vi "Delete Line.vi"(8 "error in":errorcluster, 10 "Active Line Name":string, 11 "dds configuration in":refnum<class "DDS configuration.lvclass">) -> (0 "error out":errorcluster, 2 "deleted line":T1, 3 "dds configuration out":refnum<class "DDS configuration.lvclass">)   [LabVIEW 2014, in "DDS configuration.lvclass"]
uses:
  DDS configuration.lvclass
  Line.ctl
  <vilib>/NI/Tag Bus Module Framework/channel/TBM channel.lvclass
  <vilib>/RTI DDS Toolkit for LabVIEW/Types/RTI DDS Advanced Reader Configuration.ctl
  DDS configuration.lvclass/DDS configuration.ctl
  <vilib>/RTI DDS Toolkit for LabVIEW/Library/LVDDS_library.lvlib
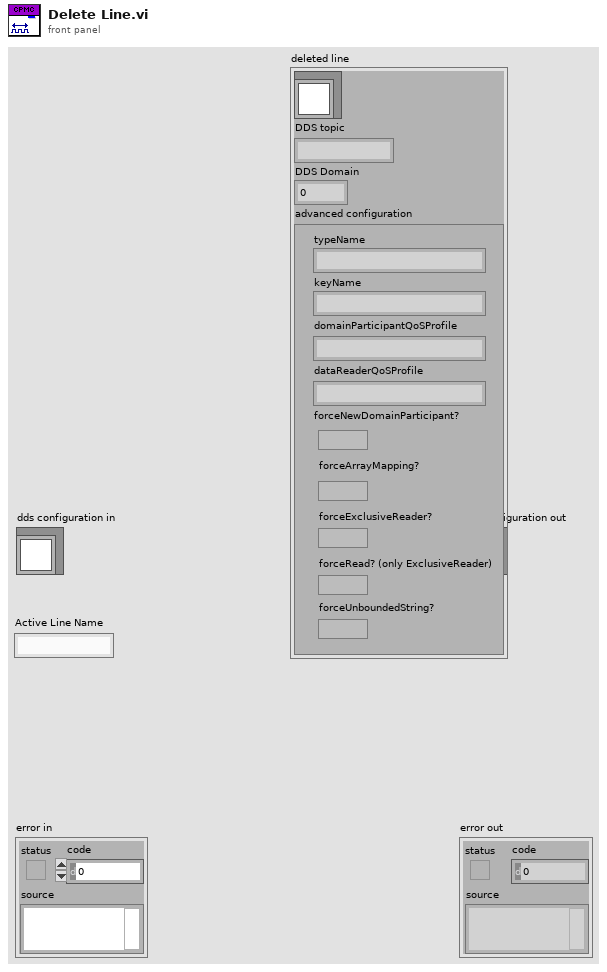
[diagram p1: front panel]
types:
  T1 = typedef "DDS configuration.lvclass/Line.ctl" = cluster{"channel":refnum<class "TBM channel.lvclass">, "DDS topic":string, "DDS Domain":u32, "advanced configuration":T2}
  T2 = typedef "LVDDS_library.lvlib/RTI DDS Advanced Reader Configuration.ctl" = cluster{"typeName":string, "keyName":string, "domainParticipantQoSProfile":string, "dataReaderQoSProfile":string, "forceNewDomainParticipant?":bool, "forceArrayMapping?":bool, "forceExclusiveReader?":bool, "forceRead? (only ExclusiveReader)":bool, "forceUnboundedString?":bool}
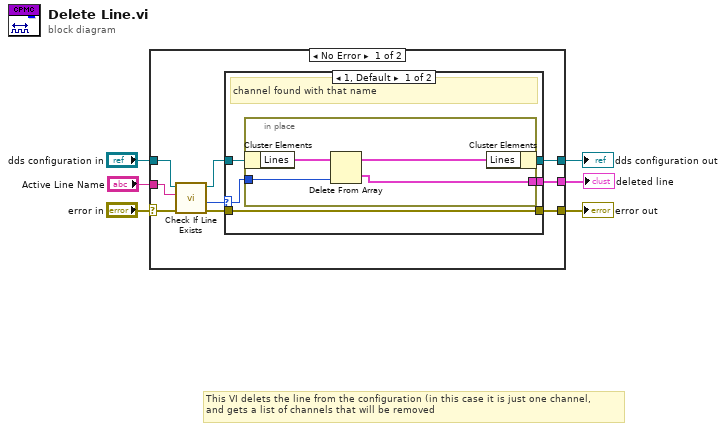
[diagram p0: block diagram]
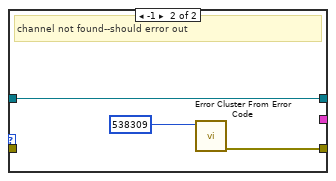
[diagram p2: hidden frame]
diagram:
  # "This VI delets the line from the configuration (in this case it is just one channel, \nand gets a list of channels that will be removed"
  n1 = case shown="No Error" "error in" {
    selector: "error in" -> [w9 w28]
    tunnel: [w15 w28] -> w6
    tunnel: [w14 w29] -> w5
    tunnel: "dds configuration in" -> [w12 w29]
    tunnel: "Active Line Name" -> [w13 _]
    tunnel: [w8 _] -> w1
    frame No Error {
      n2 = call-dynamic "Check If Line Exists.vi"("error in"=w9, "name to locate"=w13, "dds configuration in"=w12) -> ("error out"=w10:errorcluster, "index"=w7:i32, "dds configuration out"=w11:refnum<class "DDS configuration.lvclass">)  [unwired: 4 in, 2 out]
      n3 = case shown="1, Default" w7 {
        selector: w7 -> [w16 _]
        tunnel: [w18 w27] -> w15
        tunnel: w11 -> [w20 w25]
        tunnel: [w19 w25] -> w14
        tunnel: w10 -> [w18 _]
        tunnel: [w17 _] -> w8
        frame 1, Default {
          # "channel found with that name"
          n4 = in-place {
            in-place-border: w16 -> [w24]
            in-place-border: [w21] -> w17
            n5 = in-place-cluster #1(w20) -> ("Lines"=w23:T1[])
            n6 = Delete From Array(array=w23, index=w24) -> (deleted portion=w21:T1, array with subset deleted=w22:T1[])  [unwired: 1 in]
            n7 = in-place-cluster #1("Lines"=w22) -> (w19:refnum<class "DDS configuration.lvclass">)
          }
        }
        frame -1 {
          # "channel not found--should error out"
          n8 = call <vilib>:"Error Cluster From Error Code.vi"("error code (0)"=538309) -> ("error out"=w27:errorcluster)  [unwired: 8 in]
        }
      }
    }
    frame Error {
    }
  }
  "error out" <- w6
  "dds configuration out" <- w5
  "deleted line" <- w1
